vi "2.数据每秒记录一次每分钟存储为一份文件.vi"() -> ()   [LabVIEW 2018]
uses:
  <vilib>/Platform/TimedLoop/XDataNode/timing_clust.ctl
  <vilib>/Platform/TimedLoop/XDataNode/nitl_modes.ctl
  <vilib>/Platform/TimedLoop/XDataNode/wakeup.ctl
  <vilib>/Platform/TimedLoop/XDataNode/XDataNode.xnode
  <vilib>/Platform/TimedLoop/XDataNode/XDNodeRunTimeDep.lvlib
panel:
  in  "表格控件":string[][](table)
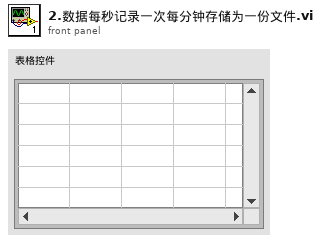
[diagram p1: front panel]
types:
  T1 = typedef "XDNodeRunTimeDep.lvlib/timing_clust.ctl" = cluster{"Expected End [f-1]":u64, "Actual End [f-1]":u64, "Finished Late? [f-1]":bool, "Expected End [i-1]":u64, "Actual End [i-1]":u64, "Finished Late? [i-1]":bool, "Expected Start [i]":u64, "Actual Start [i]":u64, "Expected Start [f]":u64, "Actual Start [f]":u64, "Source Name":string, "Structure Name":string, "Period":i64, "Deadline":i64, "Offset":i64, "Start":i64, "Priority":i32, "Timeout":i32, "Mode":T2, "Wakeup Reason":T3, "Error":errorcluster, "Source Type":string, "Secondary Source Type":string, "Global End Time":u64, "Global Start Time":u64, "Frame Duration":u64, "Iteration Duration":u64, "Assigned CPU":i32, "I/O Scan Engine Mode":u32}
  T2 = typedef "XDNodeRunTimeDep.lvlib/nitl_modes.ctl" = enum32{"No Change", "Process missed periods, maintain original phase", "Discard missed periods, maintain original phase", "Process missed periods, ignore original phase", "Discard missed periods, ignore original phase"}
  T3 = typedef "XDNodeRunTimeDep.lvlib/wakeup.ctl" = enum32{"Normal", "Aborted", "Asynchronous wakeup", "Timing source error", "Timed loop error", "Timeout"}
  T4 = enum16{"open", "replace", "create", "open or create", "replace or create", "replace or create with confirmation"}
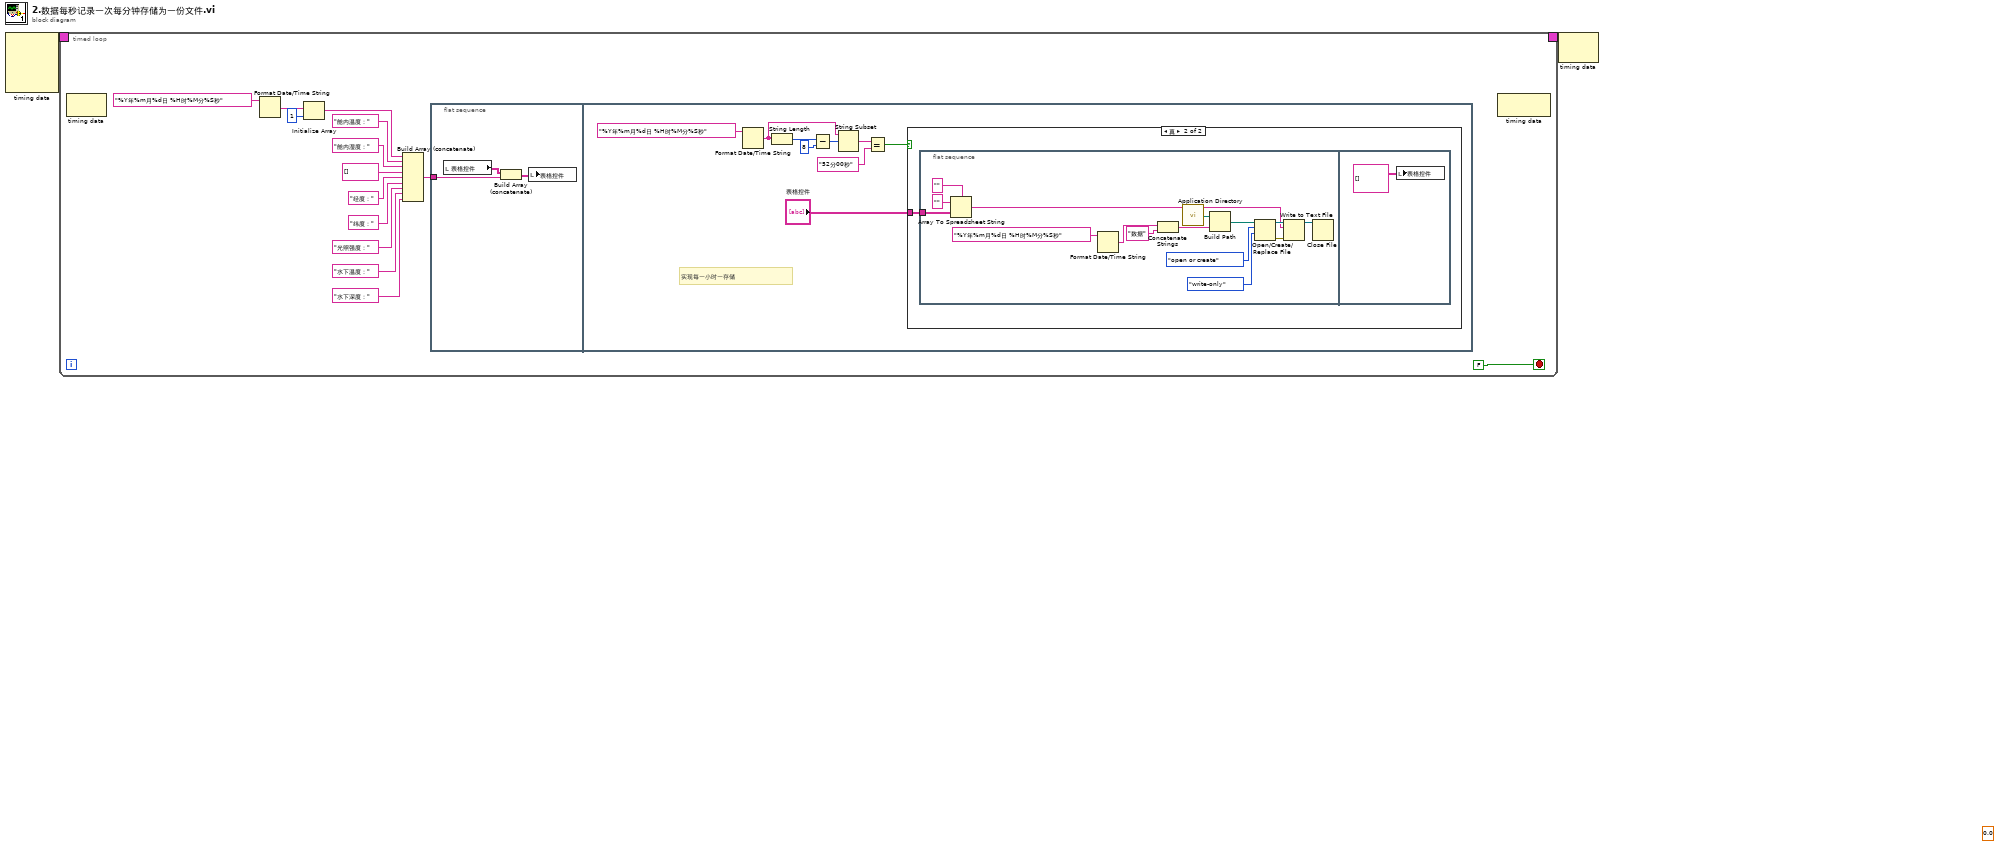
[diagram p0: block diagram]
diagram:
  (unwired) 0.0 ("水下深度")
  n1 = node-c288() -> (w2:T1)  [unwired: 4 in]
  n2 = timed-loop {
    timing: w2 -> [_]
    timing-out: [_] -> w1
    stop <- FALSE stop-if-true
    n3 = node-c288() -> ()  [unwired: 1 in, 1 out]
    n4 = Format Date/Time String(time format string (%c)="%Y年%m月%d日 %H时%M分%S秒" ("时间格式字符串(%c)")) -> (date/time string=w15:string)  [unwired: 2 in]
    n5 = Initialize Array(w15, 1 ("维数大小")) -> (w13:string[])
    n6 = Build Array (concatenate)(w13, "舱内温度：", "舱内湿度：", string[] [] ("元素"), "经度：", "纬度：", "光照强度：", "水下温度：", "水下深度：") -> (w12:string[])
    n7 = flat-sequence {
      tunnel: w12 -> [w19]
      frame #0 {
        n8 = local read "表格控件"() -> (w18:string[][])
        n9 = Build Array (concatenate)(w18, w19) -> (w17:string[][])
        n10 = local write "表格控件"(w17) -> ()
      }
      frame #1 {
        # "实现每一小时一存储"
        n11 = Format Date/Time String(time format string (%c)="%Y年%m月%d日 %H时%M分%S秒" ("时间格式字符串(%c)")) -> (date/time string=w27:string)  [unwired: 2 in]
        n12 = String Length(string=w27) -> (length=w26:i32)
        n13 = Subtract(x=w26, y=8) -> (x-y=w24:i32)
        n14 = String Subset(string=w27, offset (0)=w24) -> (substring=w23:string)  [unwired: 1 in]
        n15 = Equal?(x=w23, y="52分00秒") -> (x = y?=w21:bool)
        n16 = case shown="真" w21 {
          tunnel: "表格控件" -> [_ w29]
          frame False {
          }
          frame True {
            n17 = flat-sequence {
              tunnel: w29 -> [w42]
              frame #0 {
                n18 = Array To Spreadsheet String(delimiter (Tab)="" ("分隔符(Tab)"), array=w42, 3:"" ("格式字符串")) -> (spreadsheet string=w31:string)
                n19 = Format Date/Time String(time format string (%c)="%Y年%m月%d日 %H时%M分%S秒" ("时间格式字符串(%c)")) -> (date/time string=w40:string)  [unwired: 2 in]
                n20 = Concatenate Strings(w40, "数据" ("字符串")) -> (w39:string)
                n21 = call <vilib>:"Application Directory.vi"() -> ("Application Directory"=w30:path)
                n22 = Build Path(base path=w30, name or relative path=w39) -> (appended path=w36:path)
                n23 = Open/Create/Replace File(file path (use dialog)=w36, operation (0:open)=T4."open or create" ("操作(0:open)"), access (0:read/write)=enum16{"read/write", "read-only", "write-only"}."write-only" ("权限(0:read/write)")) -> (refnum out=w37:refnum<file>, error out=w38:errorcluster)  [unwired: 3 in, 1 out]
                n24 = Write to Text File(file (use dialog)=w37, text=w31, error in=w38) -> (refnum out=w41:refnum<file>)  [unwired: 1 in, 2 out]
                n25 = Close File(refnum=w41) -> ()  [unwired: 1 in, 2 out]
              }
              frame #1 {
                n26 = local write "表格控件"(string[][] [] ("表格缓冲区")) -> ()
              }
            }
          }
        }
      }
    }
    n27 = node-c288() -> ()  [unwired: 1 in, 1 out]
  }
  n28 = node-c288(w1) -> ()  [unwired: 1 out]
